vi "FTW-Image-AppendToPicture.vi"(1 "Image":T1, 3 "Initial Picture":picture) -> (0 "Picture":picture)   [LabVIEW 2015]
panel:
  # "Inputs"
  # "Outputs"
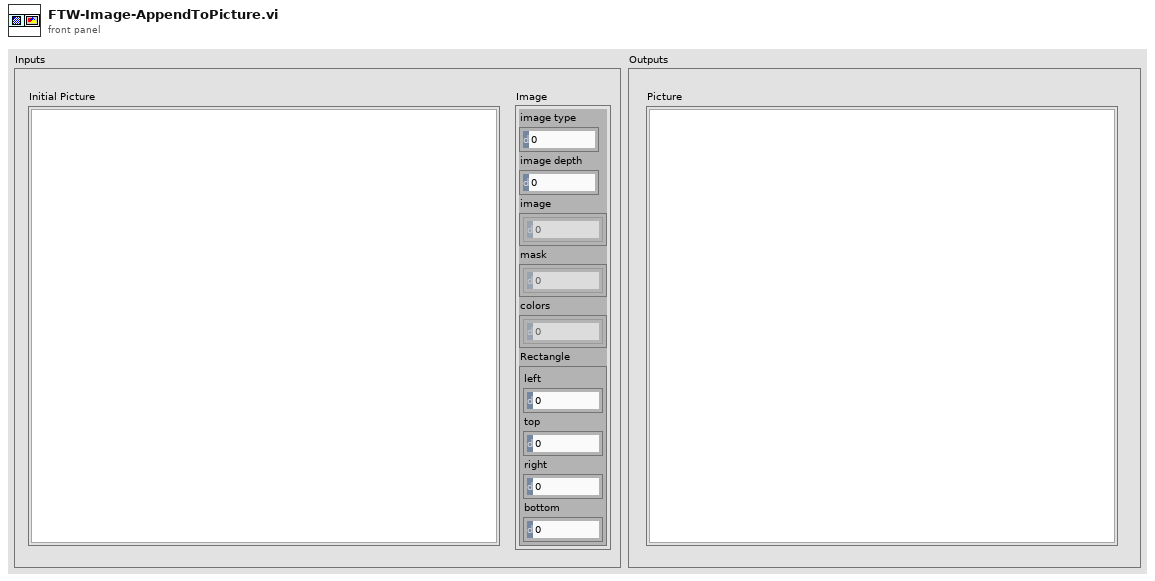
[diagram p1: front panel]
types:
  T1 = cluster{"image type":i32, "image depth":i32, "image":u8[], "mask":u8[], "colors":u32[], "Rectangle":cluster{"left":i16, "top":i16, "right":i16, "bottom":i16}}
  T2 = cluster{"Copy Pixmap opcode":i16, i32, i32, "top":i16, "left":i16, i16, i16, "Bits per pixel":i16, "default foreground":u32, "default background":u32, "No color table; use default RGB":u16}
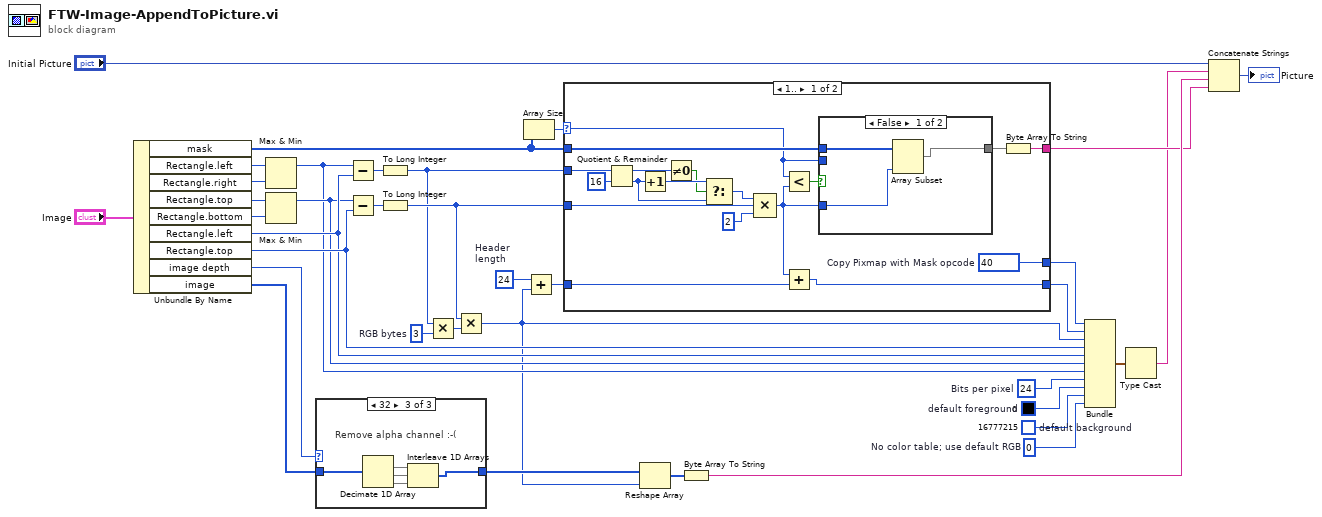
[diagram p0: block diagram]
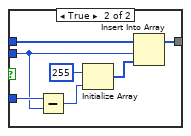
[diagram p2: hidden frame]
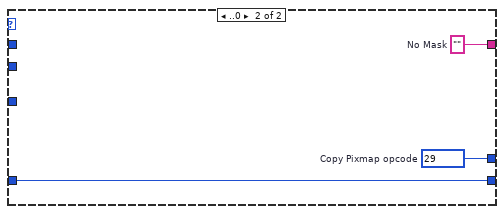
[diagram p3: hidden frame]
diagram:
  w6 = 24  # Header length
  w10 = u16 0  # No color table; use default RGB
  w16 = i16 24  # Bits per pixel
  w22 = u32 16777215  # default background
  w23 = u32 0  # default foreground
  w19 = 3  # RGB bytes
  n1 = Unbundle By Name("Image") -> ("mask"=w15:u8[], "Rectangle.left"=w30:i16, "Rectangle.right"=w29:i16, "Rectangle.top"=w28:i16, "Rectangle.bottom"=w27:i16, "Rectangle.left"=w13:i16, "Rectangle.top"=w14:i16, "image depth"=w32:i32, "image"=w31:u8[])
  n2 = Max & Min(x=w30, y=w29) -> (max(x,y)=w11:i16)  [unwired: 1 out]
  n3 = Max & Min(x=w28, y=w27) -> (max(x,y)=w12:i16)  [unwired: 1 out]
  n4 = case shown="32" w32 {
    tunnel: w31 -> [_ w37 w42]
    tunnel: [_ w37 w38] -> w18
    frame Default {
    }
    frame 24 {
    }
    frame 32 {
      # "Remove alpha channel :-("
      n5 = Decimate 1D Array(w42) -> (w41:u8[], w40:u8[], w39:u8[])  [unwired: 1 out]
      n6 = Interleave 1D Arrays(w41, w40, w39) -> (w38:u8[])
    }
  }
  n7 = Subtract(x=w11, y=w13) -> (x-y=w35:i16)
  n8 = Subtract(x=w12, y=w14) -> (x-y=w34:i16)
  n9 = To Long Integer(number=w35) -> (32bit integer=w8:i32)
  n10 = To Long Integer(number=w34) -> (32bit integer=w9:i32)
  n11 = Multiply(x=w8, y=w19) -> (x*y=w20:i32)
  n12 = Multiply(x=w9, y=w20) -> (x*y=w7:i32)
  n13 = Array Size(array=w15) -> (size(s)=w21:i32)
  n14 = Add(x=w6, y=w7) -> (x+y=w5:i32)
  n15 = case shown="1.." w21 {
    selector: w21 -> [w55 _]
    tunnel: w9 -> [w60 _]
    tunnel: [w52 w72] -> w4
    tunnel: [w57 w73] -> w33
    tunnel: w15 -> [w56 _]
    tunnel: [w51 w71] -> w26
    tunnel: w8 -> [w45 _]
    tunnel: w5 -> [w54 w72]
    frame 1.. {
      w51 = i16 40  # Copy Pixmap with Mask opcode
      n16 = Quotient & Remainder(x=w45, y=16) -> (x-y*floor(x/y)=w48:i32, floor(x/y)=w50:i32)
      n17 = Increment(x=w50) -> (x+1=w49:i32)
      n18 = Not Equal To 0?(x=w48) -> (x != 0?=w47:bool)
      n19 = Select(t=w49, s=w47, f=w50) -> (s? t:f=w43:i32)
      n20 = Compound Arithmetic op=MULTIPLY(w43, w60, 2 ("y")) -> (w53:i32)
      n21 = Less?(x=w55, y=w53) -> (x < y?=w59:bool)
      n22 = Add(x=w53, y=w54) -> (x+y=w52:i32)
      n23 = case shown="False" w59 {
        tunnel: w56 -> [w63 w67]
        tunnel: w55 -> [_ w66]
        tunnel: w53 -> [w62 w70]
        tunnel: [w61 w65] -> w58
        frame False {
          n24 = Array Subset(array=w63, length=w62) -> (w61:u8[])  [unwired: 1 in]
        }
        frame True {
          n25 = Subtract(x=w70, y=w66) -> (x-y=w69:i32)
          n26 = Initialize Array(u8 255 ("element"), w69) -> (w68:u8[])
          n27 = Insert Into Array(array=w67, index=w66, new element=w68) -> (w65:u8[])
        }
      }
      n28 = Byte Array To String(unsigned byte array=w58) -> (string=w57:string)
    }
    frame ..0 {
      w71 = i16 29  # Copy Pixmap opcode
      w73 = ""  # No Mask
    }
  }
  n29 = Reshape Array(w18, w7) -> (w17:u8[])
  n30 = Byte Array To String(unsigned byte array=w17) -> (string=w36:string)
  n31 = Bundle("Copy Pixmap opcode"=w26, w4, w7, "top"=w14, "left"=w13, w12, w11, "Bits per pixel"=w16, "default foreground"=w23, "default background"=w22, "No color table; use default RGB"=w10) -> (w25:T2)  [unwired: 1 in]
  n32 = Type Cast(x=w25) -> (*(type *) &x=w24:string)  [unwired: 1 in]
  n33 = Concatenate Strings("Initial Picture", w24, w36, w33) -> (→"Picture":picture)
